vi "CLD 7 Time Stamp to String Challenge Exercise.vi"(8 "Error In":errorcluster) -> (0 "Error Out":errorcluster, 3 "Code String Out":string)   [LabVIEW 2025]
doc: "CLD 7 exercise"
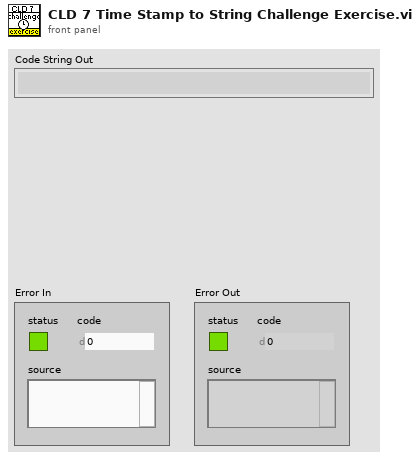
[diagram p1: front panel]
types:
  T1 = typedef "LVDateTimeRec.ctl" = cluster{"fractional second":dbl, "second":i32, "minute":i32, "hour":i32, "day of month":i32, "month":i32, "year":i32, "day of week":i32, "day of year":i32, "DST":i32}
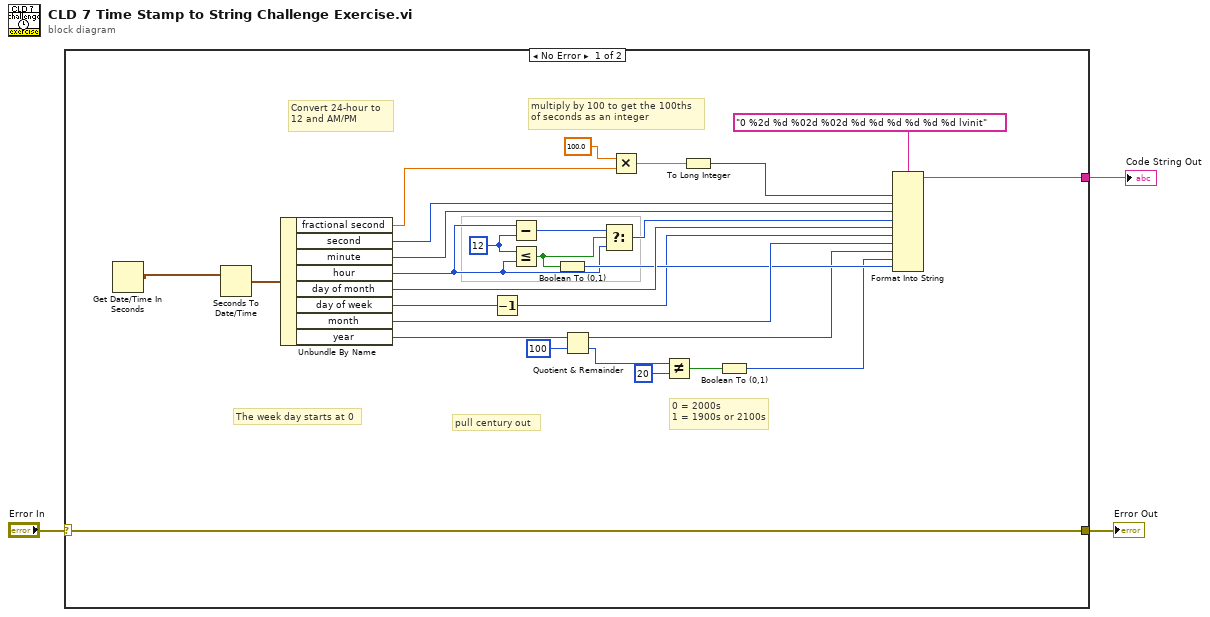
[diagram p0: block diagram]
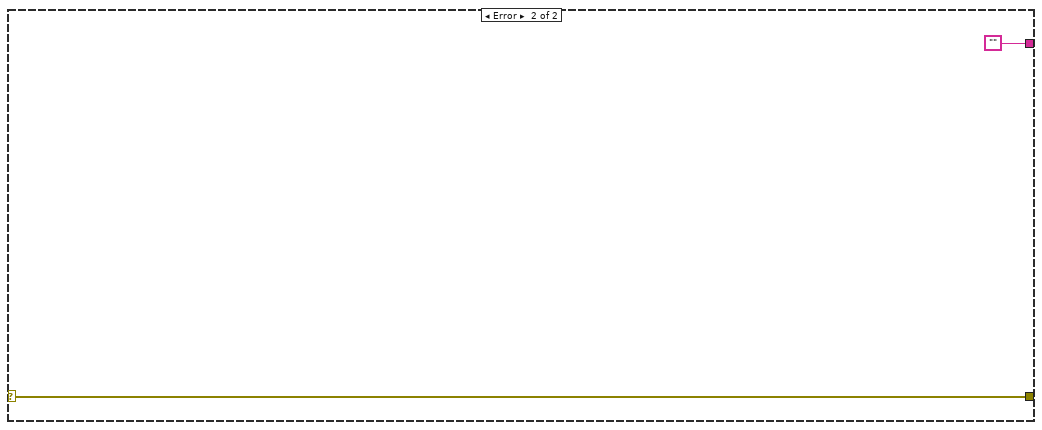
[diagram p2: hidden frame]
diagram:
  n1 = case shown="No Error" "Error In" {
    selector: "Error In" -> [w31 w33]
    tunnel: [w31 w33] -> w2
    tunnel: [w28 ""] -> w1
    frame No Error {
      w18 = 12 ("y")
      # "The week day starts at 0"
      # "Convert 24-hour to\n12 and AM/PM"
      # "multiply by 100 to get the 100ths\nof seconds as an integer"
      # "0 = 2000s\n1 = 1900s or 2100s"
      # "pull century out"
      n2 = Get Date/Time In Seconds() -> (seconds since 1Jan1904=w16:timestamp)
      n3 = Seconds To Date/Time(time stamp (now)=w16) -> (date time rec=w30:T1)  [unwired: 1 in]
      n4 = Unbundle By Name(w30) -> ("fractional second"=w27:dbl, "second"=w25:i32, "minute"=w24:i32, "hour"=w12:i32, "day of month"=w23:i32, "day of week"=w22:i32, "month"=w21:i32, "year"=w10:i32)
      n5 = Decrement(x=w22) -> (x-1=w11:i32)
      n6 = Subtract(x=w12, y=w18) -> (x-y=w19:i32)
      n7 = Less Or Equal?(x=w18, y=w12) -> (x <= y?=w13:bool)
      n8 = Boolean To (0,1)(Boolean=w13) -> (0, 1=w20:i16)
      n9 = Quotient & Remainder(x=w10, y=100) -> (x-y*floor(x/y)=w8:i32, floor(x/y)=w7:i32)
      n10 = Select(t=w19, s=w13, f=w12) -> (s? t:f=w17:i32)
      n11 = Multiply(x=100.0 ("y"), y=w27) -> (x*y=w15:dbl)
      n12 = Not Equal?(x=w7, y=20) -> (x != y?=w5:bool)
      n13 = To Long Integer(number=w15) -> (32bit integer=w14:i32)
      n14 = Boolean To (0,1)(Boolean=w5) -> (0, 1=w4:i16)
      n15 = Format Into String(format string="0 %2d %d %02d %02d %d %d %d %d %d %d lvinit", w14, w25, w24, w17, w23, w11, w21, w8, w4, w20) -> (resulting string=w28:string)  [unwired: 2 in, 1 out]
    }
    frame Error {
    }
  }
  "Code String Out" <- w1
  "Error Out" <- w2
